vi "Comm Command Engine.vi"(6 "Loop Time (ms)":u32=10, 8 "error in (no error)":errorcluster, 10 "Comm.lvclass":refnum<class "VeriStand Comm.lvclass">, 11 "Process":refnum<class "Process.lvclass">) -> (0 "error out":errorcluster)   [LabVIEW 2018, in "NI VeriStand Addon Network Comm.lvlib" / "VeriStand Comm.lvclass"]
uses:
  VeriStand Comm.lvclass
  <vilib>/NI/NIVS Inline Async API/_VS Inline Async API/Process/Process.lvclass
  VeriStand Comm.lvclass/VeriStand Comm.ctl
  <vilib>/NI/STM/TCP/TCP Read Options.ctl
  <vilib>/NI/STM/Connection Manager/TCP/TCP Connection Method.ctl
  Shared/_Types/Comm Message.ctl
  <vilib>/NI/STM/TCP/TCP Write Options.ctl
  <vilib>/NI/NIVS Inline Async API/_VS Inline Async API/Process/Process.lvclass/Process.ctl
  <vilib>/NI/STM/TCP/Get Connection Reference (TCP).vi
  <vilib>/NI/AMC/Create Single Message.vi
  <vilib>/NI/AMC/Update Message Routing Info.vi
  <vilib>/NI/Tools/Keyed Array/Map String.vi
  <vilib>/NI/AMC/Read Termination Message.vi
  <vilib>/NI/NIVS Inline Async API/_VS Inline Async API/Error Handling Process/SubVIs/Error.ConvertArray.vi
  <vilib>/NI/STM/SubVIs/Generate STM Error.vi
  <vilib>/NI/Tools/String/Get Case Matching.vi
  <vilib>/NI/STM/TCP/Read Message (TCP).vi
  <vilib>/NI/AMC/Send Message.vi
  Shared/Comm Constants.vi
  <vilib>/NI/AMC/Globals.vi
  <vilib>/NI/STM/TCP/Write Message (TCP).vi
  <vilib>/NI Veristand/Custom Device Tools/Custom Device Utility Library/Custom Device Utility Library.lvlib
  <vilib>/NI/Tools/Keyed Array/Tools_KeyedArray.lvlib
  <vilib>/NI/AMC/AMC.lvlib
  <vilib>/NI/STM/NI STM.lvlib
  Shared/NI VeriStand Addon Network Comm Shared.lvlib
  <vilib>/Utility/SystemLogging/NI_SystemLogging.lvlib
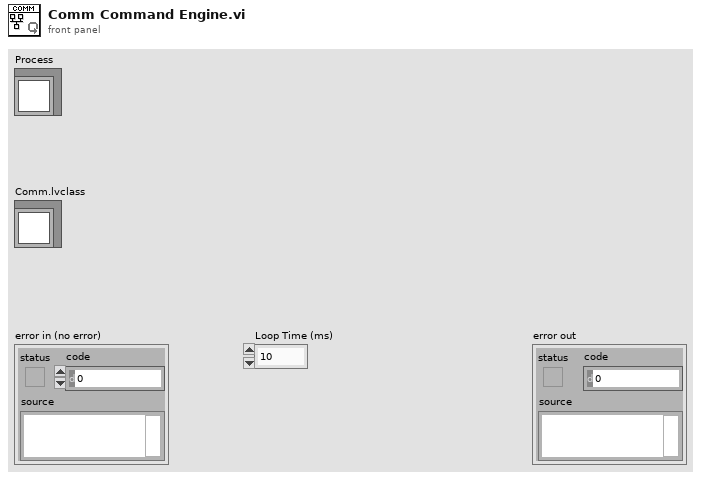
[diagram p1: front panel]
types:
  T1 = typedef "NI STM.lvlib/TCP Read Options.ctl" = cluster{"ignore timeout error":bool, "timeout ms (1000)":i32}
  T2 = typedef "AMC.lvlib/Message Queue.ctl" = refnum<queue>
  T3 = typedef "NI STM.lvlib/TCP Connection Manager Reference.ctl" = refnum<data-value>
  T4 = typedef "NI STM.lvlib/TCP Connection Method.ctl" = enum16{"Initialize", "Add Connection", "Set Properties", "Get Connection(s)", "Remove Connection", "Remove All Connections", "Get Connection Count"}
  T5 = typedef "NI VeriStand Addon Network Comm Shared.lvlib/Comm Message.ctl" = cluster{"Timeout":u32, "Resp?":bool, "data":string}
  T6 = typedef "NI STM.lvlib/TCP Write Options.ctl" = cluster{"ignore timeout error":bool, "timeout ms (1000)":i32}
  T7 = typedef "NI STM.lvlib/TCP Connection Info.ctl" = cluster{"connection ID":refnum<k5>, "meta data":T8[]}
  T8 = typedef "NI STM.lvlib/MetaDataElement.ctl" = string
  T9 = typedef "Tools_KeyedArray.lvlib/KeyedArray.ctl" = cluster{"keys":string[], "values":string[]}
  T10 = typedef "NI STM.lvlib/TCP Connection Properties.ctl" = cluster{"Name":string, "Address":string, "Custom":string}
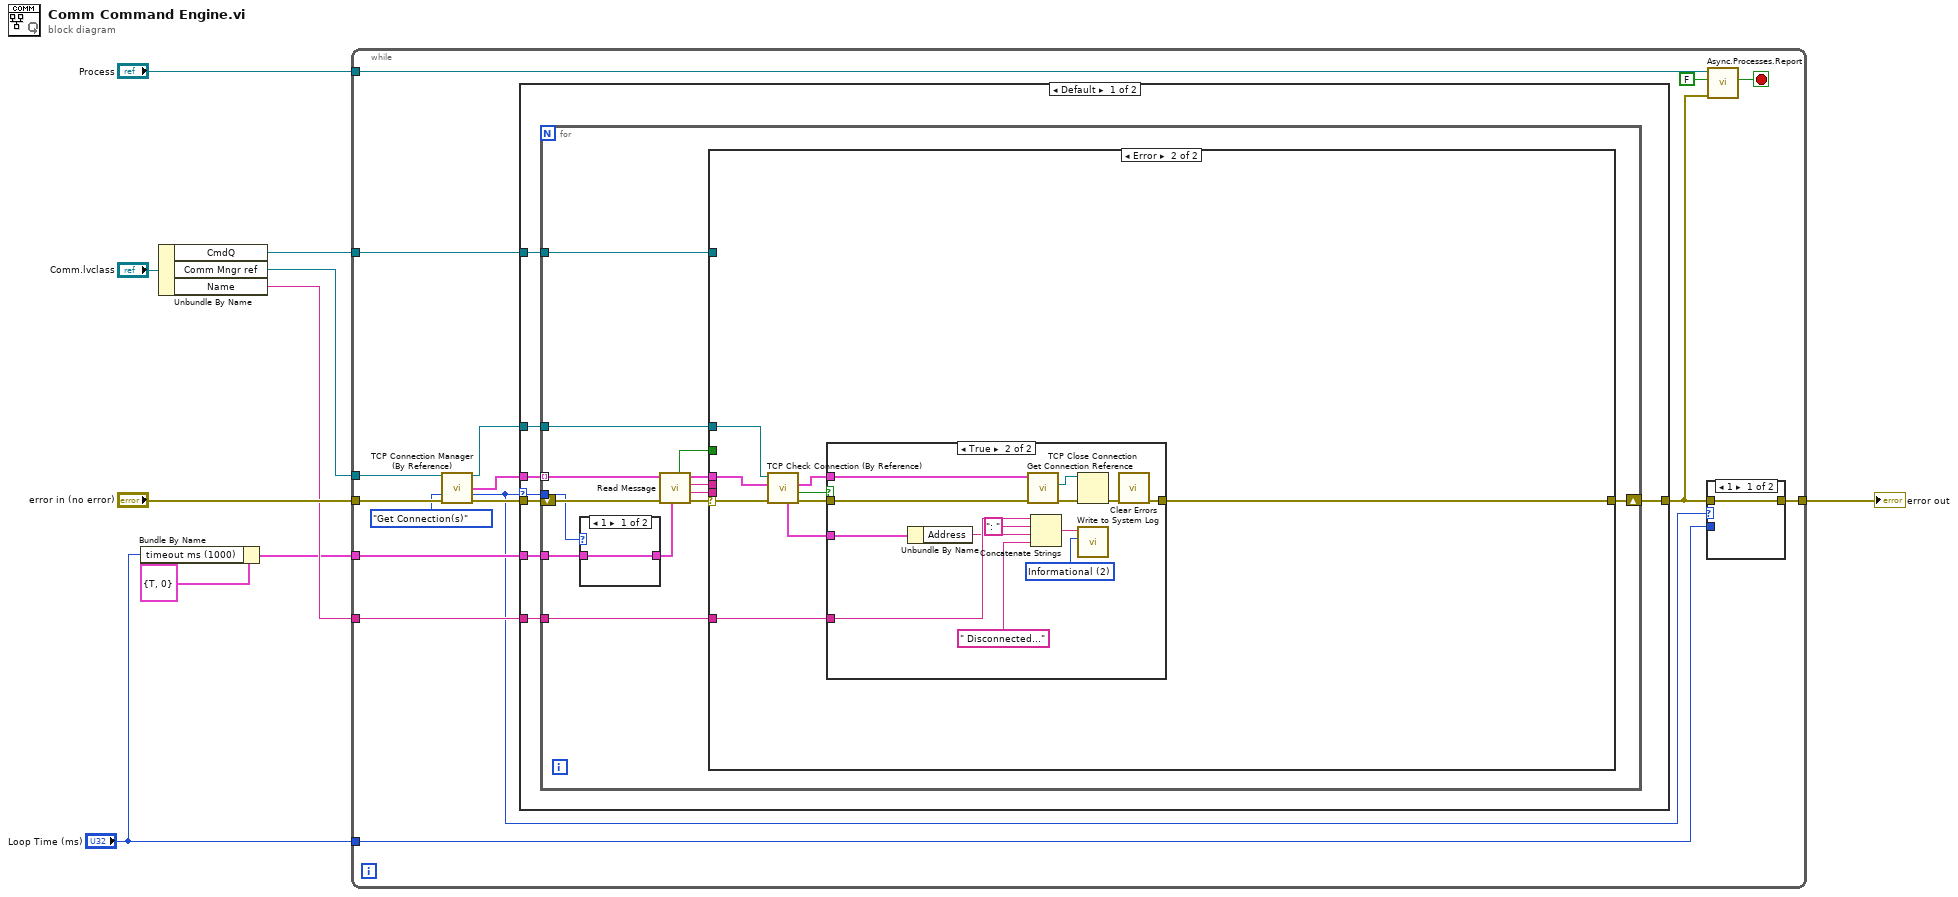
[diagram p0: block diagram]
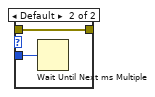
[diagram p2: hidden frame]
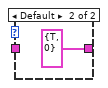
[diagram p3: hidden frame]
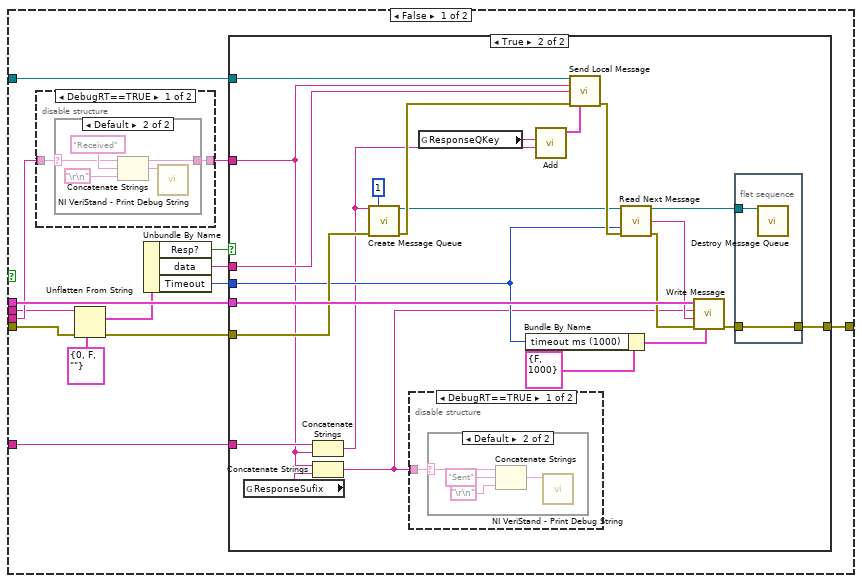
[diagram p5: hidden frame]
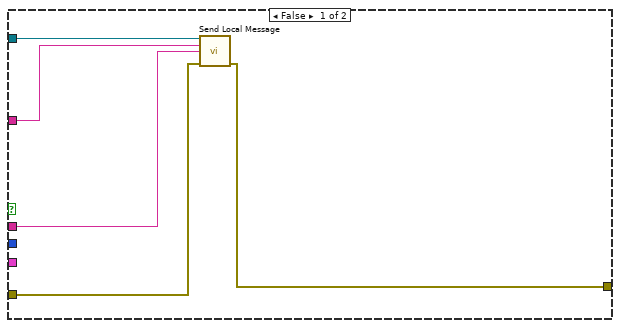
[diagram p8: hidden frame]
diagram:
  n1 = Bundle By Name(cluster=T1 {"ignore timeout error"=TRUE, "timeout ms (1000)"=0} ("options"), "timeout ms (1000)"="Loop Time (ms)") -> (w1:T1)
  n2 = Unbundle By Name("Comm.lvclass") -> ("CmdQ"=w5:T2, "Comm Mngr ref"=w9:T3, "Name"=w6:string)
  n3 = while {
    tunnel: "error in (no error)" -> [w26]
    tunnel: [w13] -> w7
    tunnel: w9 -> [w23]
    tunnel: "Process" -> [w20]
    tunnel: w6 -> [w22]
    tunnel: w5 -> [w21]
    tunnel: "Loop Time (ms)" -> [w16]
    tunnel: w1 -> [w14]
    stop <- w18 stop-if-true
    n4 = call <vilib>:"TCP Connection Manager (By Reference).vi"("connection manager ref in"=w23, "method"=TCP_Connection_Method."Get Connection(s)", "error in"=w26) -> ("connection manager ref out"=w24:T3, "all connections"=w15:T7[], "number of connections"=w11:i32, "error out"=w25:errorcluster)  [unwired: 6 in, 3 out]
    n5 = case shown="Default" w11 {
      selector: w11 -> [w31 _]
      tunnel: w15 -> [w37 _]
      tunnel: w25 -> [w33 w143]
      tunnel: w24 -> [w36 _]
      tunnel: [w35 w143] -> w12
      tunnel: w22 -> [w34 _]
      tunnel: w21 -> [w32 _]
      tunnel: w14 -> [w30 _]
      frame Default {
        n6 = for {
          tunnel: w37 -> [w46] mode=indexing
          tunnel: w36 -> [w51]
          shift-right: [w50] -> w35
          shift-left: w33 -> [w48]
          tunnel: w34 -> [w49]
          tunnel: w32 -> [w41]
          tunnel: w31 -> [w39]
          tunnel: w30 -> [w38]
          n7 = case shown="1" w39 {
            tunnel: [w52 T1 {"ignore timeout error"=TRUE, "timeout ms (1000)"=0} ("options")] -> w40
            tunnel: w38 -> [w52 _]
            frame 1 {
            }
            frame Default {
            }
          }
          n8 = call-poly <vilib>:"Read Message.vi"("options"=w40, "error in"=w48, "connection info in"=w46) -> ("error out"=w47:errorcluster, "name"=w43:T8, "data string"=w44:string, "connection info out"=w45:T7, "timed out?"=w42:bool)  [unwired: 3 in, 1 out]
          n9 = case shown="Error" w47 {
            selector: w47 -> [w61 w123]
            tunnel: w51 -> [_ w125]
            tunnel: w45 -> [w54 w124]
            tunnel: [w60 w122] -> w50
            tunnel: w49 -> [w55 w121]
            tunnel: w44 -> [w59 _]
            tunnel: w43 -> [w58 _]
            tunnel: w42 -> [w57 _]
            tunnel: w41 -> [w56 _]
            frame No Error {
              n10 = case shown="True" w57 {
                tunnel: w61 -> [w64 w119]
                tunnel: [w75 w119] -> w60
                tunnel: w59 -> [w63 _]
                tunnel: w58 -> [w71 _]
                tunnel: w56 -> [w74 _]
                tunnel: w55 -> [w73 _]
                tunnel: w54 -> [w72 _]
                frame False {
                  n11 = disable-structure shown="DebugRT==TRUE" {
                    disable-tunnel: w71 -> [w77 w83]
                    disable-tunnel: [w76 w83] -> w62
                    frame condition #0 {
                      n12 = case shown="Default" w77 {
                        selector: w77 -> [w78 w79]
                        tunnel: [w78 w79] -> w76
                        frame "" {
                        }
                        frame Default {
                          n13 = Concatenate Strings(w79, "Received" ("string"), "\r\n") -> (w82:string)
                          n14 = call <vilib>:"NI VeriStand - Print Debug String.vi"("Message"=w82) -> ()  [unwired: 10 in, 1 out]
                        }
                      }
                    }
                    frame condition #1 (active) {
                    }
                  }
                  n15 = Unflatten From String(type=T5 {"Timeout"=0, "Resp?"=FALSE, "data"=""}, binary string=w63, error in (no error)=w64) -> (value=w68:T5, error out=w70:errorcluster)  [unwired: 2 in, 1 out]
                  n16 = Unbundle By Name(w68) -> ("Resp?"=w65:bool, "data"=w67:string, "Timeout"=w66:u32)
                  n17 = case shown="True" w65 {
                    tunnel: [w85 w92] -> w75
                    tunnel: w74 -> [w88 w111]
                    tunnel: w73 -> [_ w110]
                    tunnel: w72 -> [_ w109]
                    tunnel: w70 -> [w86 w105]
                    tunnel: w67 -> [w87 w104]
                    tunnel: w66 -> [_ w101]
                    tunnel: w62 -> [w84 w91]
                    frame False {
                      n18 = call <vilib>:"Send Local Message.vi"("message queue in"=w88, "message name"=w84, "message value"=w87, "error in"=w86) -> ("error out"=w85:errorcluster)  [unwired: 9 in, 2 out]
                    }
                    frame True {
                      n19 = global read "Comm Constants.vi" "ResponseSufix"() -> (w89:string)
                      n20 = Concatenate Strings(w110, w91) -> (w97:string)
                      n21 = Concatenate Strings(w91, w89) -> (w98:string)
                      n22 = call <vilib>:"Create Message Queue.vi"("message queue name"=w97, "max queue size (-1, unlimited)"=1, "error in"=w105) -> ("message queue out"=w106:T2, "error out"=w108:errorcluster)  [unwired: 11 in]
                      n23 = disable-structure shown="DebugRT==TRUE" {
                        disable-tunnel: w98 -> [w112 _]
                        frame condition #0 {
                          n24 = case shown="Default" w112 {
                            selector: w112 -> [_ w114]
                            frame "" {
                            }
                            frame Default {
                              n25 = Concatenate Strings(w114, "Sent" ("string"), "\r\n") -> (w116:string)
                              n26 = call <vilib>:"NI VeriStand - Print Debug String.vi"("Message"=w116) -> ()  [unwired: 10 in, 1 out]
                            }
                          }
                        }
                        frame condition #1 (active) {
                        }
                      }
                      n27 = global read "Comm Constants.vi" "ResponseQKey"() -> (w90:string)
                      n28 = Bundle By Name(cluster=T6 {"ignore timeout error"=FALSE, "timeout ms (1000)"=1000} ("options"), "timeout ms (1000)"=w101) -> (w93:T6)
                      n29 = call <vilib>:"Add.vi"("value"=w97, "key"=w90) -> ("array out"=w96:T9)  [unwired: 3 in, 2 out]
                      n30 = call <vilib>:"Send Local Message.vi"("message queue in"=w111, "message name"=w91, "message value"=w104, "error in"=w108, "message attributes"=w96) -> ("error out"=w107:errorcluster)  [unwired: 8 in, 2 out]
                      n31 = call <vilib>:"Read Next Message.vi"("message queue in"=w106, "timeout (1 ms)"=w101, "error in"=w107) -> ("message queue out"=w100:T2, "message value"=w102:string, "error out"=w103:errorcluster)  [unwired: 5 in, 5 out]
                      n32 = call-poly <vilib>:"Write Message.vi"("options"=w93, "error in"=w103, "data"=w102, "name"=w98, "connection info in"=w109) -> ("error out"=w99:errorcluster)  [unwired: 5 in, 1 out]
                      n33 = flat-sequence {
                        tunnel: w100 -> [w118]
                        tunnel: w99 -> [w117]
                        tunnel: [w117] -> w92
                        frame #0 {
                          n34 = call <vilib>:"Destroy Message Queue.vi"("message queue in"=w118) -> ()  [unwired: 12 in, 3 out]
                        }
                      }
                    }
                  }
                }
                frame True {
                }
              }
            }
            frame Error {
              n35 = call <vilib>:"TCP Check Connection (By Reference).vi"("error in"=w123, "connection in"=w124, "connection manager ref in"=w125) -> ("error out"=w128:errorcluster, "disconnected?"=w126:bool, "connection out"=w127:T7, "properties out"=w120:T10)  [unwired: 4 in, 1 out]
              n36 = case shown="True" w126 {
                tunnel: [w129 w139] -> w122
                tunnel: w128 -> [w129 w142]
                tunnel: w127 -> [_ w137]
                tunnel: w121 -> [_ w134]
                tunnel: w120 -> [_ w135]
                frame False {
                }
                frame True {
                  w132 = 2 items=["Error", "Warning", "Informational"] ("severity")
                  n37 = Unbundle By Name(w135) -> ("Address"=w130:string)
                  n38 = call-poly <vilib>:"Get Connection Reference.vi"("error in"=w142, "connection info in"=w137) -> ("error out"=w141:errorcluster, "connection ID out"=w140:refnum<k5>)  [unwired: 7 in, 1 out]
                  n39 = Concatenate Strings(w134, ": " ("string"), w130, " Disconnected..." ("string")) -> (w136:string)
                  n40 = TCP Close Connection(connection ID=w140, error in (no error)=w141) -> (error out=w138:errorcluster)  [unwired: 1 in, 1 out]
                  n41 = call <vilib>:"Write to System Log.vi"("severity"=w132, "message"=w136) -> ()  [unwired: 9 in, 1 out]
                  n42 = call <vilib>:"Clear Errors.vi"("error in (no error)"=w138) -> ("error out"=w139:errorcluster)  [unwired: 5 in, 1 out]
                }
              }
            }
          }
        }
      }
      frame 0 {
      }
    }
    n43 = case shown="1" w11 {
      tunnel: w16 -> [_ w29]
      tunnel: [w27 w28] -> w13
      tunnel: w12 -> [w27 w28]
      frame 1 {
      }
      frame Default {
        n44 = Wait Until Next ms Multiple(millisecond multiple=w29) -> ()  [unwired: 1 out]
      }
    }
    n45 = call <vilib>:"Async.Processes.Report.vi"("Error"=w12, "Stop Async on Error?"=FALSE ("Stop on Error?"), "Process in"=w20) -> ("Stop"=w18:bool)  [unwired: 7 in, 1 out]
  }
  "error out" <- w7
